vi "Sensor Data.vi"   [LabVIEW 2021, in "Lake Shore 336.lvlib"]
uses:
  <instrlib>/Lake Shore 336/Lake Shore 336.lvlib
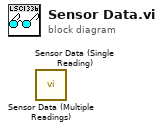
[diagram p0: block diagram]
diagram:
  n1 = call <instrlib>:"Sensor Data (Multiple Readings).vi"() -> ()  [unwired: 9 in, 3 out]
  n2 = call <instrlib>:"Sensor Data (Single Reading).vi"() -> ()  [unwired: 9 in, 3 out]
